vi "Boolean.vi"(1 "Boolean In":bool) -> (0 "Boolean out":bool)   [LabVIEW 2010]
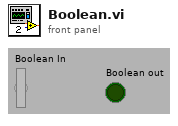
[diagram p1: front panel]
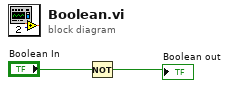
[diagram p0: block diagram]
diagram:
  n1 = Not(x="Boolean In") -> (.not. x?=→"Boolean out":bool)
